vi "CTS_RTSLoopBack.vi"(3 "error in (no error)":errorcluster {"code" format="%.0x"}, 4 "topology name":T1="2566/16-SPDT", 5 "PXI resource name":refnum<k15>="PXI1Slot6", 6 "VISA resource name":refnum<visa-resource-name>="COM1") -> (0 "error out":errorcluster, 1 "Receive_buffer":u8[](array[numeric]) format="%x", 2 "VISA resource name Out":refnum<visa-resource-name>)   [LabVIEW 2014]
uses:
  <instrlib>/niSwitch/niswitch.llb/niSwitch Topologies.ctl
panel:
  out "Read Count 2":u32
  out "Receive_buffer 2":u8[](array[numeric]) format="%x"
  out "Read Count":u32
  out "Write Count":u32
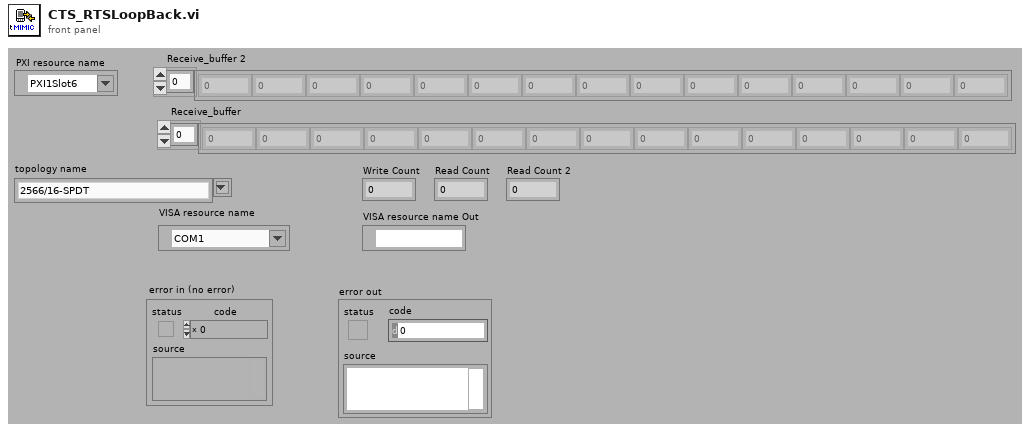
[diagram p1: front panel]
types:
  T1 = typedef "niSwitch Topologies.ctl" = string
  T2 = enum16{"Init Control Relays", "Secondary RS232", "Term Loopback", "CTS Isolate", "Synapse Loopback", "CST RTS Loopback", "Command Flash", "Auxillary RS232", "Battery Charge", "Remote Power", "Cordless Boot", "Auxillary Port", "DeInit Control Relays"}
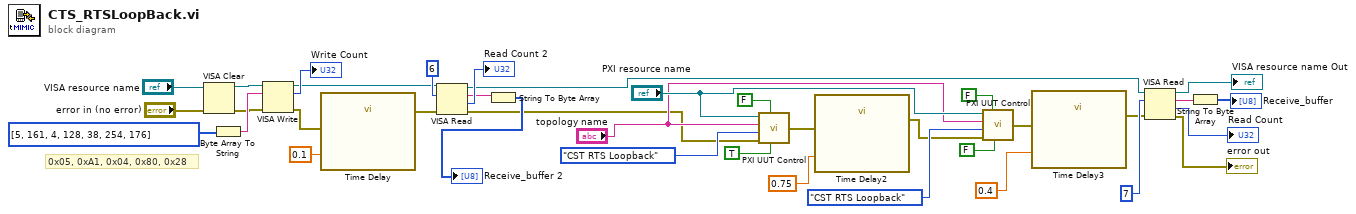
[diagram p0: block diagram]
diagram:
  # "0x05, 0xA1, 0x04, 0x80, 0x28"
  n1 = VISA Clear(VISA resource name="VISA resource name", error in (no error)="error in (no error)") -> (VISA resource name out=w17:refnum<visa-resource-name>, error out=w18:errorcluster)
  n2 = Byte Array To String(unsigned byte array=u8[] [5, 161, 4, 128, 38, 254, 176] ("Command array")) -> (string=w35:string)
  n3 = VISA Write(VISA resource name=w17, write buffer=w35, error in (no error)=w18) -> (VISA resource name out=w12:refnum<visa-resource-name>, return count=→"Write Count":u32, error out=w9:errorcluster)
  n4 = call "Time Delay"("error in (no error)"=w9, "Delay Time (s)"=0.1) -> ("error out"=w8:errorcluster)  [unwired: 9 in]
  n5 = VISA Read(VISA resource name=w12, byte count=u32 6, error in (no error)=w8) -> (VISA resource name out=w11:refnum<visa-resource-name>, read buffer=w14:string, return count=→"Read Count 2":u32, error out=w10:errorcluster)
  n6 = String To Byte Array(string=w14) -> (unsigned byte array=→"Receive_buffer 2":u8[])
  n7 = call "PXI UUT Control.vi"("Enable Relays"=TRUE, "Reset IO"=FALSE, "error in (no error)"=w10, "Enum"=T2."CST RTS Loopback", "topology name"="topology name", "resource name"="PXI resource name") -> ("error out"=w6:errorcluster)
  n8 = call "Time Delay2"("error in (no error)"=w6, "Delay Time (s)"=0.75) -> ("error out"=w5:errorcluster)  [unwired: 9 in]
  n9 = call "PXI UUT Control.vi"("Enable Relays"=FALSE, "Reset IO"=FALSE, "error in (no error)"=w5, "Enum"=T2."CST RTS Loopback", "topology name"="topology name", "resource name"="PXI resource name") -> ("error out"=w3:errorcluster)
  n10 = call "Time Delay3"("error in (no error)"=w3, "Delay Time (s)"=0.4) -> ("error out"=w2:errorcluster)  [unwired: 9 in]
  n11 = VISA Read(VISA resource name=w11, byte count=u32 7, error in (no error)=w2) -> (VISA resource name out=→"VISA resource name Out":refnum<visa-resource-name>, read buffer=w30:string, return count=→"Read Count":u32, error out=→"error out":errorcluster)
  n12 = String To Byte Array(string=w30) -> (unsigned byte array=→"Receive_buffer":u8[])
